vi "DuelistRole.vi"(8 "error in (no error)":errorcluster, 9 "RobotRef":refnum<class "Robot.lvclass">, 10 "Game in":refnum<class "Game.lvclass">, 11 "DuelistRole in":refnum<class "DuelistRole.lvclass">) -> (0 "error out":errorcluster, 2 "Robot out":refnum<class "Robot.lvclass">, 3 "DuelistRole out":refnum<class "DuelistRole.lvclass">)   [LabVIEW 2023, in "DuelistRole.lvclass"]
uses:
  DuelistRole.lvclass
  Robot_class/Robot.lvclass
  Game_class/Game.lvclass
  Role_class/Role.lvclass/Role.ctl
  ShootTactic_class/States.ctl
  Tacticbook_class/Tacticbook.lvclass/Tacticbook.ctl
  ShootTactic_class/ShootTactic.lvclass/ShootTactic.ctl
  Tacticbook_class/Read ShootTactic.vi
  ShootTactic_class/Read States.vi
  Tacticbook_class/Write ShootTactic.vi
  Role_class/Read Tacticbook.vi
  Role_class/Read tactic_index.vi
  Role_class/Write Tacticbook.vi
  Role_class/Write tactic_index.vi
  Tacticbook_class/Tacticbook.lvclass
  ShootTactic_class/ShootTactic.lvclass
panel:
  out "Game out":refnum<class "Game.lvclass">
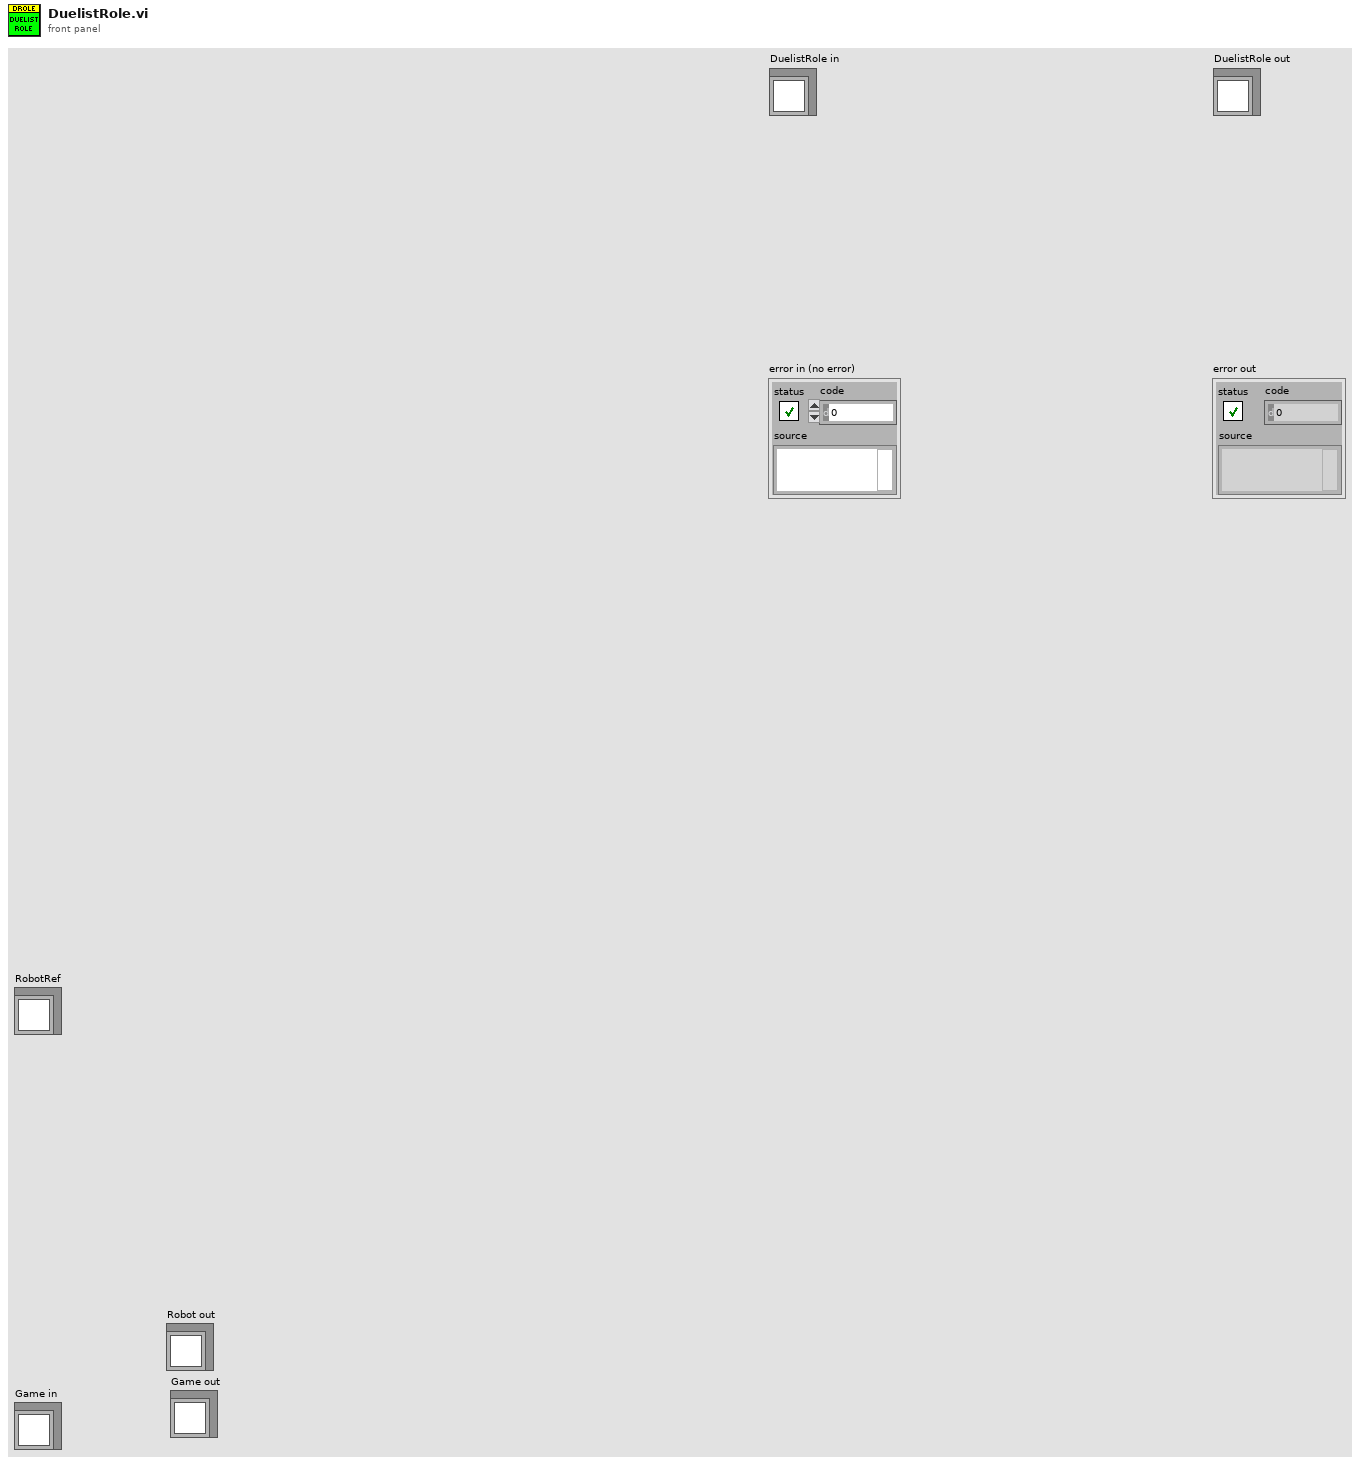
[diagram p1: front panel]
types:
  T1 = typedef "ShootTactic.lvclass/States.ctl" = enum16{"BallInGoalieArea", "Exit", "KickToGoal", "StealBall"}
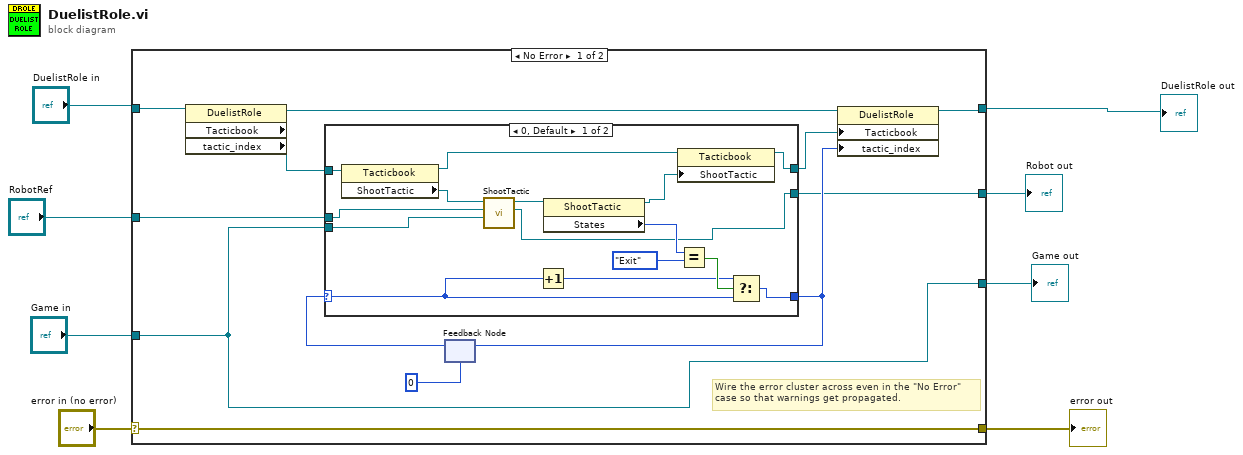
[diagram p0: block diagram]
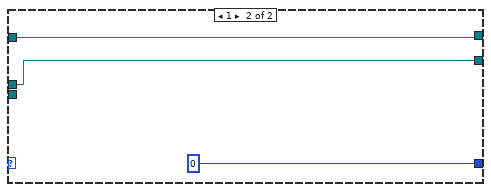
[diagram p2: hidden frame]
diagram:
  n1 = case shown="No Error" "error in (no error)" {
    selector: "error in (no error)" -> [w20 w42]
    tunnel: [w20 w42] -> w2
    tunnel: [w18 w41] -> w4
    tunnel: "DuelistRole in" -> [w19 w41]
    tunnel: "RobotRef" -> [w12 w40]
    tunnel: [w11 w40] -> w8
    tunnel: [w9 w39] -> w7
    tunnel: "Game in" -> [w9 w39]
    frame No Error {
      # "Wire the error cluster across even in the \"No Error\"\ncase so that warnings get propagated."
      n2 = property class="DuelistRole" props=["Tacticbook", "tactic_index"](reference=w19) -> (reference out=w17:refnum<class "DuelistRole.lvclass">, "Tacticbook"=w14:refnum<class "Tacticbook.lvclass">)  [unwired: 1 in, 2 out]
      n3 = feedback #1(0) -> (w15:i32)
      n4 = case shown="0, Default" w15 {
        selector: w15 -> [w32 _]
        tunnel: [w33 0] -> w13
        tunnel: w14 -> [w35 w36]
        tunnel: w12 -> [w23 w38]
        tunnel: [w24 w38] -> w11
        tunnel: [w29 w36] -> w10
        tunnel: w9 -> [w22 _]
        frame 0, Default {
          n5 = property class="Tacticbook"(reference=w35) -> (reference out=w30:refnum<class "Tacticbook.lvclass">, "ShootTactic"=w28:refnum<class "ShootTactic.lvclass">)  [unwired: 1 in, 1 out]
          n6 = call "ShootTactic.vi"("Game in"=w22, "Robot"=w23, "ShootTactic in"=w28) -> ("Robot out"=w24:refnum<class "Robot.lvclass">, "ShootTactic out"=w27:refnum<class "ShootTactic.lvclass">)  [unwired: 6 in, 1 out]
          n7 = Increment(x=w32) -> (x+1=w31:i32)
          n8 = property class="ShootTactic"(reference=w27) -> (reference out=w26:refnum<class "ShootTactic.lvclass">, "States"=w25:T1)  [unwired: 1 in, 1 out]
          n9 = property class="Tacticbook"(reference=w30, "ShootTactic"=w26) -> (reference out=w29:refnum<class "Tacticbook.lvclass">)  [unwired: 1 in, 1 out]
          n10 = Equal?(x=w25, y=States."Exit") -> (x = y?=w34:bool)
          n11 = Select(t=w31, s=w34, f=w32) -> (s? t:f=w33:i32)
        }
        frame 1 {
        }
      }
      n12 = feedback-in #1(w13) -> ()
      n13 = property class="DuelistRole"(reference=w17, "Tacticbook"=w10, "tactic_index"=w13) -> (reference out=w18:refnum<class "DuelistRole.lvclass">)  [unwired: 1 in, 1 out]
    }
    frame Error {
    }
  }
  "error out" <- w2
  "DuelistRole out" <- w4
  "Robot out" <- w8
  "Game out" <- w7
